vi "HackRF_SetGain_RxRF.vi"(8 "error in (no error)":errorcluster, 10 "AMPEnable":bool, 11 "HackRF in":T1) -> (0 "error out":errorcluster, 3 "HackRF out":T1)   [LabVIEW 2016]
doc: "RF (\"amp\", 0 or 14 dB)\n\nThe three RX gain controls are at the RF (\"amp\", 0 or 14 dB), IF gain (\"lna\", 0 to 40 dB in 8 dB steps), and baseband (\"vga\", 0 to 62 dB in 2 dB steps) stages."
uses:
  HackRF_Ref.ctl
  C:/Program Files/HackRF/labview/x64/NetHackrfx64.dll
  NetHackrfx64.dll
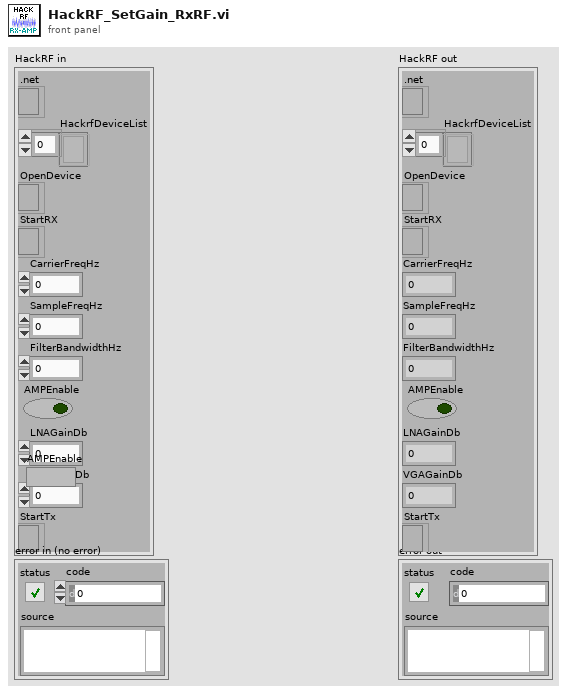
[diagram p1: front panel]
types:
  T1 = typedef "HackRF_Ref.ctl" = cluster{".net":refnum<k24>, "HackrfDeviceList":refnum<k24>[], "OpenDevice":refnum<k24>, "StartRX":refnum<k24>, "CarrierFreqHz":dbl, "SampleFreqHz":dbl, "FilterBandwidthHz":dbl, "AMPEnable":bool, "LNAGainDb":dbl, "VGAGainDb":dbl, "StartTx":refnum<k24>}
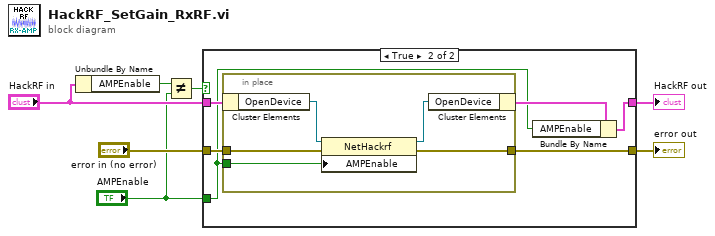
[diagram p0: block diagram]
diagram:
  n1 = Unbundle By Name("HackRF in") -> ("AMPEnable"=w3:bool)
  n2 = Not Equal?(x=w3, y="AMPEnable") -> (x != y?=w1:bool)
  n3 = case shown="True" w1 {
    tunnel: "error in (no error)" -> [w9 w15]
    tunnel: [w9 w14] -> w6
    tunnel: [w8 w11] -> w5
    tunnel: "HackRF in" -> [w8 w13]
    tunnel: "AMPEnable" -> [_ w10]
    frame False {
    }
    frame True {
      n4 = in-place {
        in-place-border: w15 -> [w18]
        in-place-border: [w17] -> w14
        in-place-border: w10 -> [w16]
        n5 = in-place-cluster #1(w13) -> ("OpenDevice"=w20:refnum<k24>)
        n6 = property class="NetHackrf"(reference=w20, error in=w18, "AMPEnable"=w16) -> (reference out=w19:refnum<k24>, error out=w17:errorcluster)
        n7 = in-place-cluster #1("OpenDevice"=w19) -> (w12:T1)
      }
      n8 = Bundle By Name(cluster=w12, "AMPEnable"=w10) -> (w11:T1)
    }
  }
  "error out" <- w6
  "HackRF out" <- w5
